vi "Global_Sigma.vi"() -> ()   [LabVIEW 2011]
panel:
  out "AxisY_needRun?":bool
  out "AxisX_needRun?":bool
  in  "Init_PosY":dbl
  in  "Init_PosX":dbl
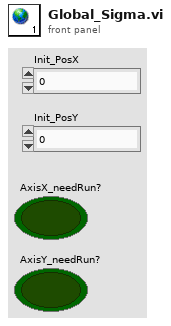
[diagram p1: front panel]
diagram:
